vi "TRIGER_LEVEL.vi"(0 "VISA resource name":refnum<visa-resource-name>="GPIB0::1::INSTR", 1 "V Unit":enum32{"mVOLT", "VOLT"}(radio), 2 "TRIGER MAIN LEVEL":string) -> ()   [LabVIEW 2018]
panel:
  # "TDS2014B"
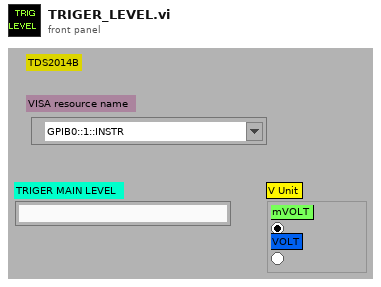
[diagram p1: front panel]
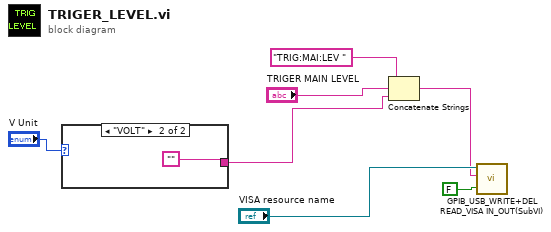
[diagram p0: block diagram]
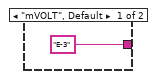
[diagram p2: hidden frame]
diagram:
  n1 = case shown="\"VOLT\"" "V Unit" {
    tunnel: ["E-3" ""] -> w1
    frame "mVOLT", Default {
    }
    frame "VOLT" {
    }
  }
  n2 = Concatenate Strings("TRIG:MAI:LEV ", "TRIGER MAIN LEVEL", w1) -> (w3:string)
  n3 = call "GPIB_USB_WRITE+DEL READ_VISA IN_OUT(SubVI).vi"("VISA resource IN"="VISA resource name", "GPIB/USB WRITE"=w3, 4:FALSE ("READ GPIB")) -> ()  [unwired: 3 in, 3 out]
